vi "Фильтрация показаний прибора.vi"(0 "Среднее":dbl, 2 "Текущее показание":dbl, 4 "Разница между \nпоказаниями прибора":u8) -> (1 "Ошибка \nприбора":bool, 7 "Отфильтрован.\nвеличина":dbl)   [LabVIEW 2013]
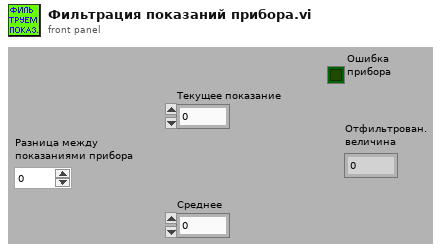
[diagram p1: front panel]
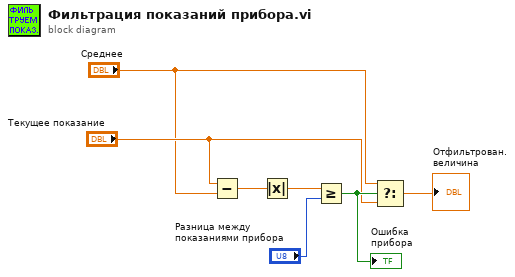
[diagram p0: block diagram]
diagram:
  n1 = Subtract(x="Текущее показание", y="Среднее") -> (x-y=w4:dbl)
  n2 = Absolute Value(x=w4) -> (abs(x)=w6:dbl)
  n3 = Greater Or Equal?(x=w6, y="Разница между \nпоказаниями прибора") -> (x >= y?=w7:bool)
  "Ошибка \nприбора" <- w7
  n4 = Select(t="Среднее", s=w7, f="Текущее показание") -> (s? t:f=→"Отфильтрован.\nвеличина":dbl)
